vi "LED_Project_LabView2015.vi"() -> ()   [LabVIEW 2011]
uses:
  <vilib>/DAQmx/write.llb/DAQmx Write (Digital Bool 1Line 1Point).vi
  <vilib>/DAQmx/create/channels.llb/DAQmx Create Channel (DO-Digital Output).vi
  <vilib>/DAQmx/miscellaneous.llb/DAQmx Fill In Error Info.vi
panel:
  out "INT_B":u32(colorbox)
  out "INT_G":u32(colorbox)
  out "INT_R":u32(colorbox)
  out "LED_B":dbl
  out "LED_G":dbl
  out "LED_R":dbl
  in  "Color Box":u32(colorbox)
  in  "COLOR BOX SWITCH":bool
  in  "BLUE":tag
  in  "GREEN":tag
  in  "REG":tag
  in  "Manual STOP":bool
  in  "LED_B":dbl(slide) scale=0.0..255.0
  in  "LED _G":dbl(slide) scale=0.0..255.0
  in  "LED_R":dbl(slide) scale=0.0..255.0
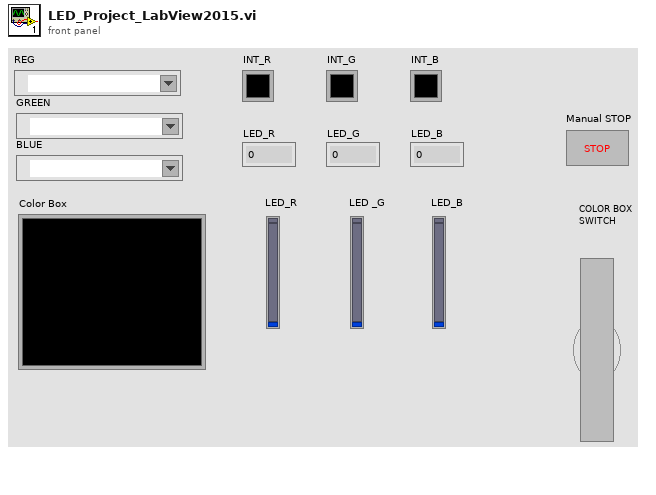
[diagram p1: front panel]
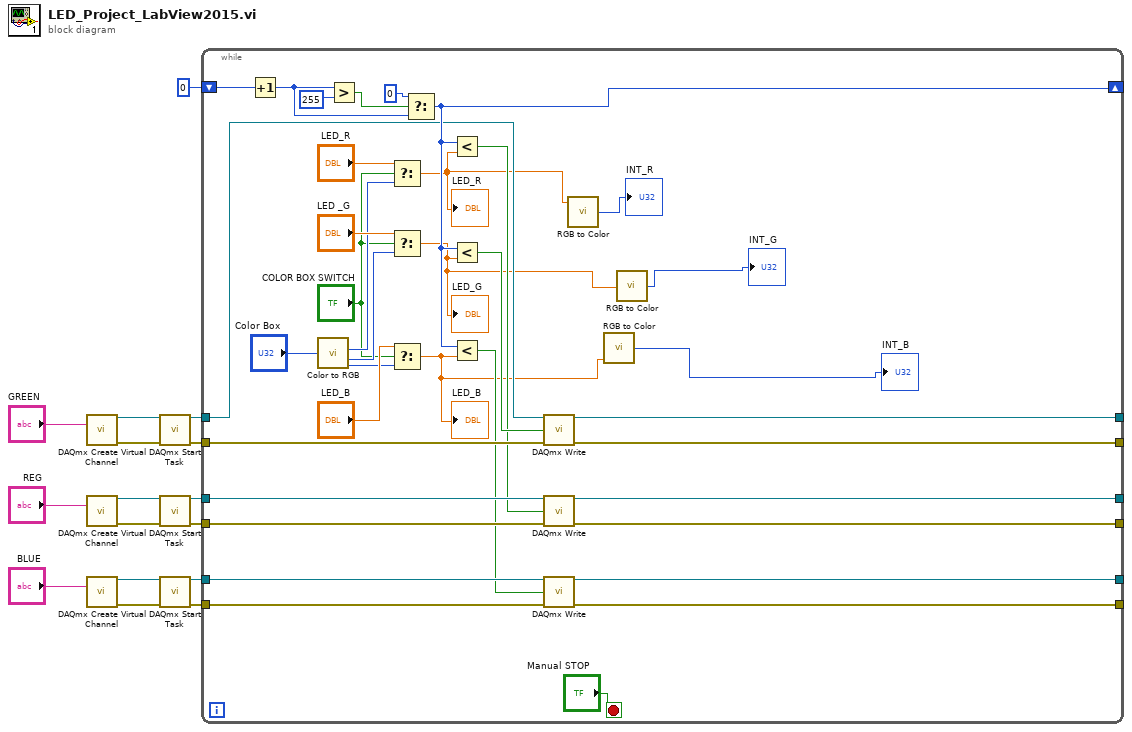
[diagram p0: block diagram]
diagram:
  n1 = call-poly <vilib>:"DAQmx Create Virtual Channel.vi"("lines"="GREEN") -> ("task out"=w15:refnum<k21>, "error out"=w14:errorcluster)  [unwired: 13 in]
  n2 = call-poly <vilib>:"DAQmx Create Virtual Channel.vi"("lines"="REG") -> ("task out"=w11:refnum<k21>, "error out"=w10:errorcluster)  [unwired: 13 in]
  n3 = call-poly <vilib>:"DAQmx Create Virtual Channel.vi"("lines"="BLUE") -> ("task out"=w7:refnum<k21>, "error out"=w6:errorcluster)  [unwired: 13 in]
  n4 = call <vilib>:"DAQmx Start Task.vi"("task/channels in"=w15, "error in"=w14) -> ("task out"=w13:refnum<k21>, "error out"=w12:errorcluster)  [unwired: 12 in]
  n5 = call <vilib>:"DAQmx Start Task.vi"("task/channels in"=w11, "error in"=w10) -> ("task out"=w9:refnum<k21>, "error out"=w8:errorcluster)  [unwired: 12 in]
  n6 = call <vilib>:"DAQmx Start Task.vi"("task/channels in"=w7, "error in"=w6) -> ("task out"=w5:refnum<k21>, "error out"=w4:errorcluster)  [unwired: 12 in]
  n7 = while {
    shift-right: [w49] -> _
    shift-left: 0 -> [w52]
    tunnel: w13 -> [w48]
    tunnel: w12 -> [w47]
    tunnel: w9 -> [w46]
    tunnel: w8 -> [w45]
    tunnel: w5 -> [w44]
    tunnel: w4 -> [w43]
    tunnel: [w42] -> _
    tunnel: [w41] -> _
    tunnel: [w40] -> _
    tunnel: [w39] -> _
    tunnel: [w38] -> _
    tunnel: [w37] -> _
    stop <- "Manual STOP" stop-if-true
    n8 = Increment(x=w52) -> (x+1=w51:i32)
    n9 = call <vilib>:"Color to RGB.vi"("Color"="Color Box") -> ("R"=w26:u8, "G"=w27:u8, "B"=w28:u8)  [unwired: 1 out]
    n10 = Greater?(x=w51, y=255) -> (0:w33:bool)
    n11 = Select(t="LED_R", s="COLOR BOX SWITCH", f=w26) -> (s? t:f=w18:dbl)
    "LED_R" <- w18
    n12 = Select(t="LED _G", s="COLOR BOX SWITCH", f=w27) -> (s? t:f=w20:dbl)
    "LED_G" <- w20
    n13 = Select(t="LED_B", s="COLOR BOX SWITCH", f=w28) -> (s? t:f=w22:dbl)
    "LED_B" <- w22
    n14 = Select(t=0, s=w33, f=w51) -> (s? t:f=w49:i32)
    n15 = Less?(x=w49, y=w18) -> (x < y?=w34:bool)
    n16 = Less?(x=w49, y=w20) -> (x < y?=w35:bool)
    n17 = Less?(x=w49, y=w22) -> (x < y?=w36:bool)
    n18 = call-poly <vilib>:"DAQmx Write.vi"("task/channels in"=w48, "data"=w35, "error in"=w47) -> ("task out"=w40:refnum<k21>, "error out"=w39:errorcluster)  [unwired: 10 in, 1 out]
    n19 = call-poly <vilib>:"DAQmx Write.vi"("task/channels in"=w46, "data"=w34, "error in"=w45) -> ("task out"=w42:refnum<k21>, "error out"=w41:errorcluster)  [unwired: 10 in, 1 out]
    n20 = call-poly <vilib>:"DAQmx Write.vi"("task/channels in"=w44, "data"=w36, "error in"=w43) -> ("task out"=w38:refnum<k21>, "error out"=w37:errorcluster)  [unwired: 10 in, 1 out]
    n21 = call <vilib>:"RGB to Color.vi"("R"=w18) -> ("Color"=→"INT_R":u32)  [unwired: 2 in]
    n22 = call <vilib>:"RGB to Color.vi"("B"=w22) -> ("Color"=→"INT_B":u32)  [unwired: 2 in]
    n23 = call <vilib>:"RGB to Color.vi"("G"=w20) -> ("Color"=→"INT_G":u32)  [unwired: 2 in]
  }
